vi "Remove UI Message Duplicates.vi"(11 "Messages In":T1[](array[typedef])) -> (3 "Messages Out":T1[](array[typedef]))   [LabVIEW 2019, in "User Interface.lvlib"]
doc: "Removes duplicate messages from the input message array, where a duplicate message is defined at the same target and event (the data value can differ). Only the newest messages are returned."
uses:
  User Interface.lvlib
  Packed Libraries/Messaging.lvlibp/Message Cluster.ctl
  Packed Libraries/Messaging.lvlibp
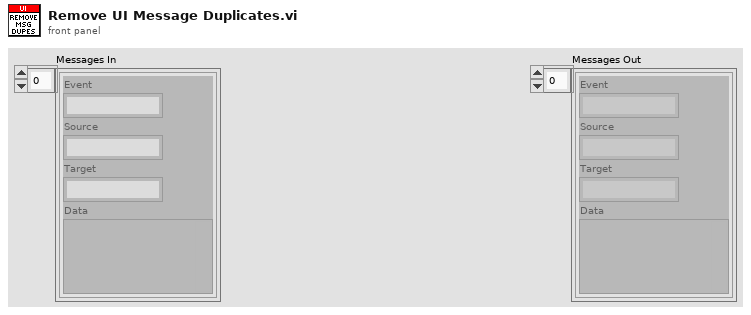
[diagram p1: front panel]
types:
  T1 = typedef "Messaging.lvlibp/Message Cluster.ctl" = cluster{"Event":string, "Source":string, "Target":string, "Data":variant}
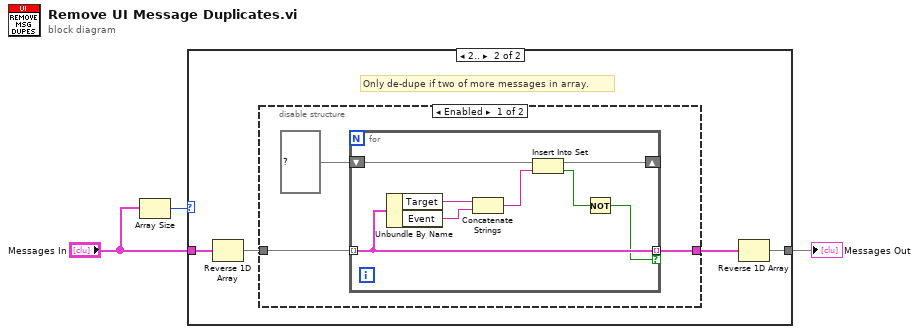
[diagram p0: block diagram]
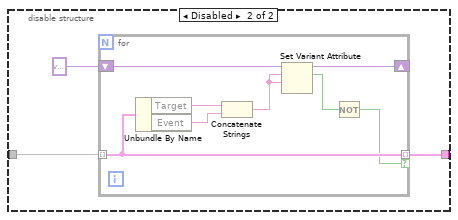
[diagram p3: hidden frame]
diagram:
  n1 = Array Size(array="Messages In") -> (size(s)=w1:i32)
  n2 = case shown="2.." w1 {
    tunnel: [w4 w7] -> w3
    tunnel: "Messages In" -> [w4 w5]
    frame Default {
      # "Zero or one message in array, nothing to de-dupe."
    }
    frame 2.. {
      # "Only de-dupe if two of more messages in array."
      n3 = Reverse 1D Array(array=w5) -> (reversed array=w8:T1[])
      n4 = disable-structure shown="Enabled" {
        disable-tunnel: w8 -> [w11 w22]
        disable-tunnel: [w9 w21] -> w6
        frame Enabled {
          n5 = for {
            tunnel: w11 -> [w13] mode=indexing
            shift-right: [w14] -> _
            shift-left: set{string} {} ("set in") -> [w16]
            tunnel: [w13] -> w9 mode=indexing if=w12
            n6 = Unbundle By Name(w13) -> ("Target"=w19:string, "Event"=w18:string)
            n7 = Concatenate Strings(w19, w18) -> (w17:string)
            n8 = Insert Into Set(10:w17, 11:w16) -> (2:w15:bool, 3:w14:set{string})
            n9 = Not(x=w15) -> (.not. x?=w12:bool)
          }
        }
        frame Disabled {
          n10 = for {
            tunnel: w22 -> [w25] mode=indexing
            shift-right: [w26] -> _
            shift-left: variant -> [w28]
            tunnel: [w25] -> w21 mode=indexing if=w24
            n11 = Unbundle By Name(w25) -> ("Target"=w30:string, "Event"=w29:string)
            n12 = Concatenate Strings(w30, w29) -> (w23:string)
            n13 = Set Variant Attribute(Variant=w28, name=w23, value=w23) -> (Variant out=w26:variant, replaced=w27:bool)  [unwired: 1 in, 1 out]
            n14 = Not(x=w27) -> (.not. x?=w24:bool)
          }
        }
      }
      n15 = Reverse 1D Array(array=w6) -> (reversed array=w7:T1[])
    }
  }
  "Messages Out" <- w3
